vi "initialize.vi"(0 "HGF_DFSMVisitor":refnum<class "HGF_DFSMVisitor.lvclass">, 3 "initializationData":variant, 5 "error in (no error)":errorcluster, 7 "binaryString":string, 8 "I8 Array":i8[](array[numeric]), 9 "prependSize? (T)":bool, 11 "byteOrder (0:big-endian, network order)":T1(ring)) -> (14 "dup HGF_DFSMVisitor":refnum<class "HGF_DFSMVisitor.lvclass">, 17 "found?":bool, 19 "error out":errorcluster)   [LabVIEW 2012, in "HGF_DeviceFSM.lvlib" / "HGF_DFSMVisitor.lvclass"]
doc: "This is a dynamic dispatch VI to be implemented by child classes to initialize their attributes.\n\n<B>Recommendation:</B> Use Variant for initialization data."
uses:
  HGF_DFSMVisitor.lvclass
  HGF_DeviceBaseClasses/HGF_DeviceVisitor/HGF_DeviceVisitor.lvclass
  HGF_DeviceFSM/HGF_DeviceFSM.lvsc/Trigger.ctl
  HGF_BaseClasses/HGF_NetworkVisitor/HGF_NetworkVisitor.lvclass
  HGF_DFSMVisitor.lvclass/HGF_DFSMVisitor.ctl
  HGF_DeviceFSM/HGF_DeviceFSM.lvsc
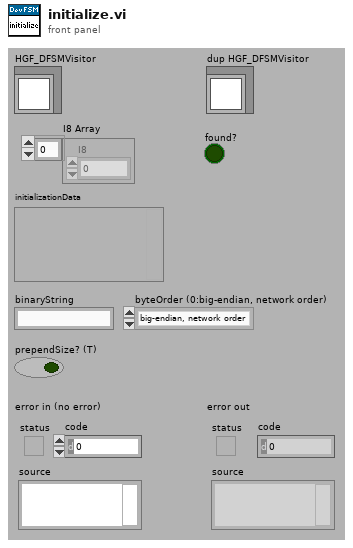
[diagram p1: front panel]
types:
  T1 = enum16{"big-endian, network order", "native, host order", "little-endian"}
  T2 = typedef "HGF_DeviceFSM.lvlib/HGF_DeviceFSM.lvsc/Trigger.ctl" = enum16{"NULL", "configure", "fault", "error", "resetError", "STOP", "visit", "not_configured", "done", "ok", "previsit", "configured"}
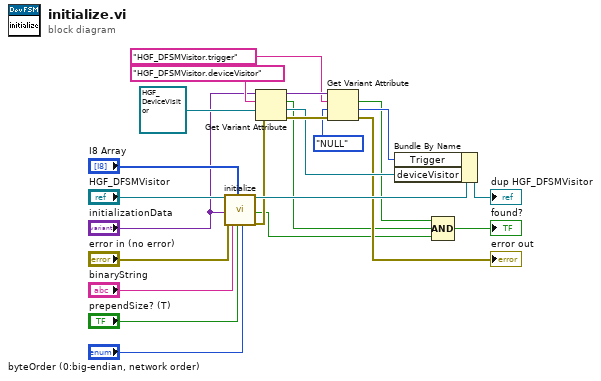
[diagram p0: block diagram]
diagram:
  n1 = call-parent "initialize.vi"("HGF_NetworkData"="HGF_DFSMVisitor", "initializationData"="initializationData", "error in (no error)"="error in (no error)", "binaryString"="binaryString", "I8 Array"="I8 Array", "prependSize? (T)"="prependSize? (T)", "byteOrder (0:big-endian, network order)"="byteOrder (0:big-endian, network order)") -> ("dup HGF_NetworkData"=w11:refnum<class "HGF_DFSMVisitor.lvclass">, "found?"=w3:bool, "error out"=w6:errorcluster)  [unwired: 10 out]
  n2 = Get Variant Attribute(Variant="initializationData", name="HGF_DFSMVisitor.deviceVisitor", default value (empty Variant)=refnum<class "HGF_DeviceVisitor.lvclass"> refnum ("deviceVisitor"), error in=w6) -> (duplicate Variant=w14:variant, found=w4:bool, value=w8:refnum<class "HGF_DeviceVisitor.lvclass">, error out=w12:errorcluster)
  n3 = Get Variant Attribute(Variant=w14, name="HGF_DFSMVisitor.trigger", default value (empty Variant)=Trigger."NULL" ("Trigger"), error in=w12) -> (found=w7:bool, value=w9:T2, error out=→"error out":errorcluster)  [unwired: 1 out]
  n4 = Bundle By Name(cluster=w11, "Trigger"=w9, "deviceVisitor"=w8) -> (→"dup HGF_DFSMVisitor":refnum<class "HGF_DFSMVisitor.lvclass">)
  n5 = Compound Arithmetic op=AND(w7, w4, w3) -> (→"found?":bool)
